vi "Global Test.vi"() -> ()   [LabVIEW 2013]
panel:
  out "Numeric":dbl
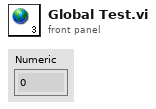
[diagram p1: front panel]
diagram:
